vi "SearchStringIntoArray.vi"(8 "error in":errorcluster, 10 "ArrayOfStringr":string[](array[string]), 11 "SearchString":string) -> (0 "error out":errorcluster, 2 "OK?":bool, 3 "Position":i32)   [LabVIEW 2013]
panel:
  out "#Found":i32
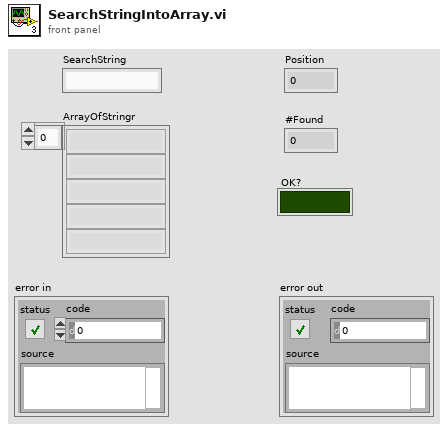
[diagram p1: front panel]
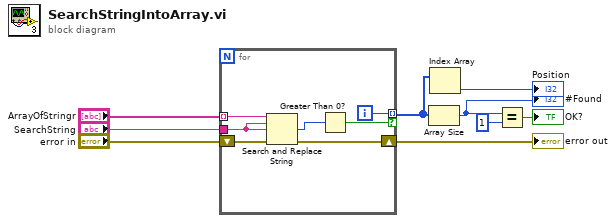
[diagram p0: block diagram]
diagram:
  n1 = for {
    tunnel: "ArrayOfStringr" -> [w16] mode=indexing
    tunnel: "SearchString" -> [w15]
    shift-right: [w14] -> w9
    shift-left: "error in" -> [w13]
    tunnel: [w11] -> w5 mode=indexing if=w10
    i -> [w11]
    n2 = Search and Replace String(input string=w16, search string=w15, replace string=w15, error in=w13) -> (number of replacements=w12:i32, error out=w14:errorcluster)  [unwired: 4 in, 2 out]
    n3 = Greater Than 0?(x=w12) -> (x > 0?=w10:bool)
  }
  "error out" <- w9
  n4 = Array Size(array=w5) -> (size(s)=w1:i32)
  "#Found" <- w1
  n5 = Index Array(array=w5) -> (element=→"Position":i32)  [unwired: 1 in]
  n6 = Equal?(x=w1, y=1) -> (x = y?=→"OK?":bool)
